vi "tdo -- V3.vi"() -> ()   [LabVIEW 2021]
uses:
  fft -- data win.ctl
  tdo -- new/Data window.ctl
  agregator -- action.ctl
  interpolation state - real.ctl
  filename-action.ctl
  <vilib>/Analysis/4window.llb/Hanning Window (DBL).vi
  <vilib>/Analysis/4window.llb/Blackman Window (DBL).vi
  linear interpolation - real -- V2.vi
  <vilib>/Analysis/4window.llb/AllCosWindow (DBL).vi
  <vilib>/Analysis/baseanly.llb/A x B.vi
  <vilib>/Analysis/baseanly.llb/Real A x B.vi
  Q -- check range -- i -- real.vi
  line -- complex.vi
  Q -- check range -- i -- integer.vi
  Q - not nan -- real.vi
  Q - not nan -- integer.vi
  <vilib>/Utility/file.llb/Write Delimited Spreadsheet (string).vi
  <vilib>/measure/matone.llb/Extract Single Tone Information 1 Chan.vi
  <vilib>/Waveform/WDTOps.llb/WDT Number of Waveform Samples DBL.vi
  <vilib>/Analysis/Matrix/Numeric/Conversions/Array To Matrix.vi
  <vilib>/Analysis/Matrix/Numeric/Conversions/Array To Matrix - RA2.vi
  <vilib>/Analysis/baseanly.llb/Inverse Matrix.vi
  <vilib>/Analysis/baseanly.llb/Real Inverse Matrix.vi
  <vilib>/Utility/file.llb/Write Delimited Spreadsheet (DBL).vi
  <vilib>/Analysis/NI_AALPro.lvlib
  <vilib>/measure/NI_MAPro.lvlib
  <vilib>/Analysis/NI_AAL_SigProc.lvlib
panel:
  in  "ccc":enum32{"Page 1", "Page 2", "Page 3"}(tab)
  in  "gamma window (sec)":dbl=0.0005 format="%#_6p"
  out "Gamma vs. Field":cluster{dbl[], dbl[]}(graph)
  out "Apmlitude or Pwr. vs. Field":cluster{dbl[], dbl[]}(graph)
  out "Frequency vs. Field":cluster{dbl[], dbl[]}(graph)
  out "Frequency vs. time":waveform(dbl)(graph)={"t0"=timestamp(-0.009969989999999984 s since 1904-01-01), "dt"=0.0001, "Y"=array[1099 elements]}
  out "Progress":dbl(slide)=0.5977589977589978 scale=0.0..1.0
  in  "aaa":enum32{"TDO settings", "file settings"}(tab)
  in  "Power spctr. threshold":dbl=0.0001 format="%.4f"
  in  "Freq. threshold":dbl=30000.0
  in  "window width (s)":dbl=0.0004 format="%#_6p"
  in  "window step (s)":dbl=0.0001 format="%#_6p"
  in  "detection method":T1(ring)
  in  "fit width":i32=9 min=3
  in  "ovewrite file?":bool
  in  "add file suffix":string="_tdo_"
  in  "remove file prefix":string="p_c4_"
  out "first line":string[](array[string])=["012_082225_time 012_082225_field 012_082225_freq 012_082225_amp 012_082225_gamma "]
  in  "Input File":path=path "/Users/arkadyshekhter/Desktop/gdrive/data/Vikram&Shiva&Zoltan--Aug2025/August_2025/082225/p_c4_012_082225.tdms"
  out "Ampl vs. time":waveform(dbl)(graph)={"t0"=timestamp(-0.009969989999999984 s since 1904-01-01), "dt"=0.0001, "Y"=array[1099 elements]}
  in  "bbb":enum32{"data settings", "Field  Settings"}(tab)
  in  "Data window":T2={"Start"=0, "Length"=1000, "Channel numbers"=[0], "Channel names"=["freq", "Field"], "Group name"="p"}
  out "dt 1":dbl=3.3e-07 format="%#_6p"
  out "dt 2":dbl=3.3e-07 format="%#_6p"
  out "Amplitude vs. Field (PWR peak)":cluster{dbl[], "Filtered X":dbl[]}(graph)
  in  "# of threads":i32=4
  out "Field profile":waveform(dbl)(graph)={"t0"=timestamp(-0.009969989999999984 s since 1904-01-01), "dt"=0.0001, "Y"=array[1099 elements]}
  # "Basic NHMFL TDO routine\nv. 0.5       F. F. Balakirev\n\nmessed with by Arkady!"
  # "Background file is either an ASCII *.dat file produced by TDO earlier\nor *.fit file containing single column of polynomial fit coeficients.\n1st row in fit file is a text header, which is ingnored. Result is saved in a \n\"*diff.dat\" file in the output folder\nExample \"PDO1.fit\": \n\nFit y=A_i*x^i, starting with A_0\n3.25637E7\n2132.56863\n-12.60591\n-2.01013\n-0.04452\n-3.23119E-4"
  # "OR"
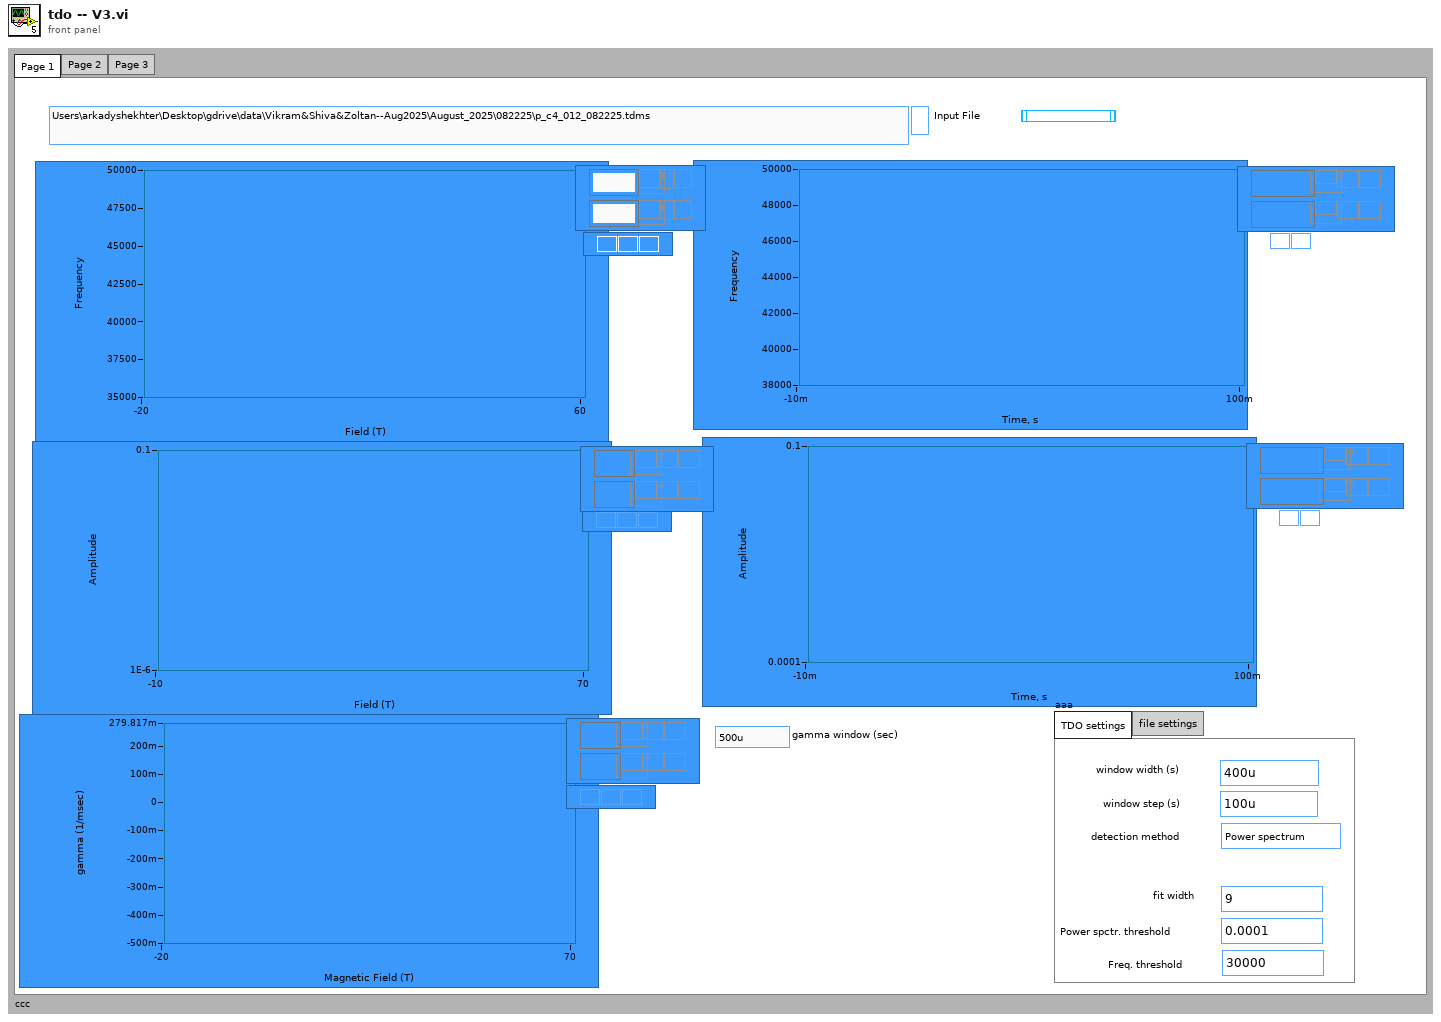
[diagram p1: front panel]
types:
  T1 = enum16{"Power spectrum", "Tone detection", "Peak-to-peak fit"}
  T2 = typedef "fft -- data win.ctl" = cluster{"Start":i64, "Length":i32, "Channel numbers":i64[], "Channel names":string[], "Group name":string}
  T3 = typedef "filename-action.ctl" = enum16{"rewrite", "parse", "force pattern", "uniquenum", "get T", "get B", "get ind", "get deg", "get name", "get folder", "get extension", "get basename", "get side", "get setof", "getID", "getIDStock", "remove prefix", "get36thing", "getplain", "getvproj", "getIDStanf"}
  T4 = typedef "interpolation state - real.ctl" = cluster{"Array ":dbl[], "actual size":i32, "requested size":i32}
  T5 = typedef "agregator -- action.ctl" = enum16{"append", "interpolate", "empty!", "force", "init", "scale", "read last"}
  T6 = typedef "Data window.ctl" = cluster{"Start":i64, "Length":i64, "Channel numbers":i64[], "Channel name":string, "Group name":string}
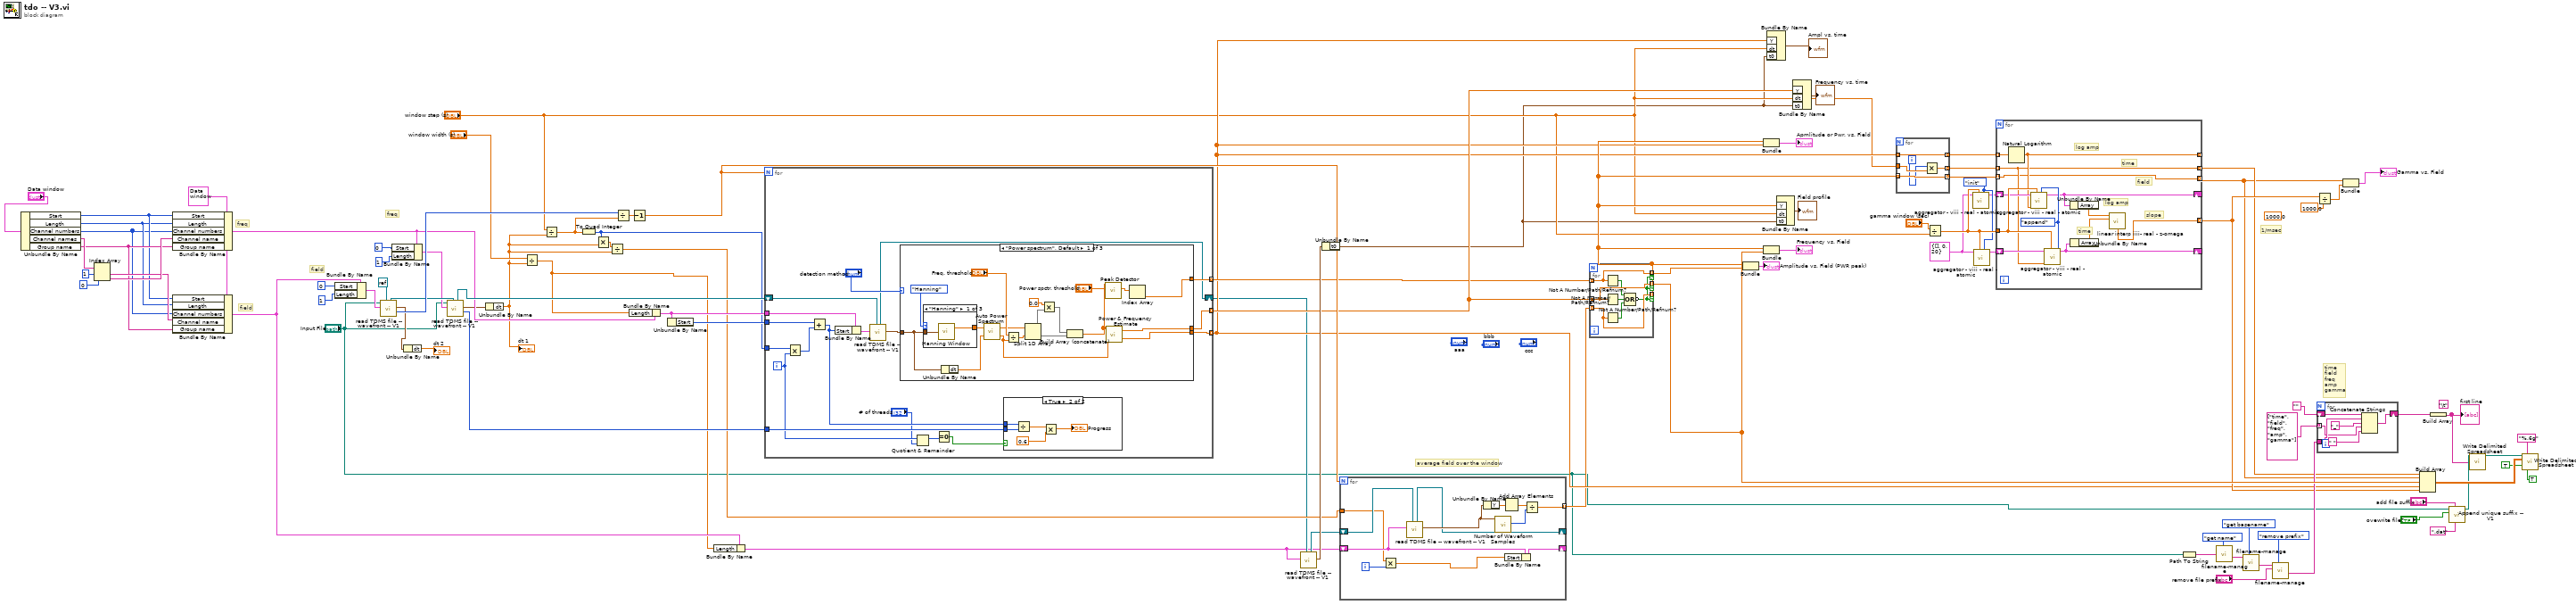
[diagram p0: block diagram]
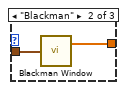
[diagram p3: hidden frame]
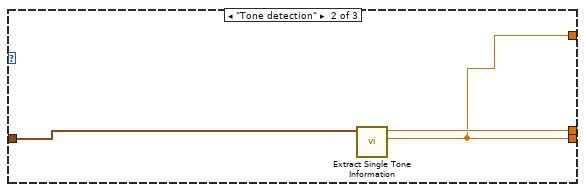
[diagram p5: hidden frame]
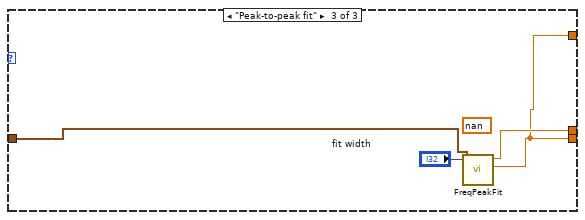
[diagram p6: hidden frame]
diagram:
  (unwired) 1000.0
  (unwired) "\t"
  w47 = T4 {"Array "=[], "actual size"=0, "requested size"=20} ("state IN")
  w51 = agregator_--_action."init" ("aggregator action")
  w14 = T6 {"Start"=0, "Length"=500000, "Channel numbers"=[0], "Channel name"="", "Group name"="Untitled"} ("Data window")
  # "average field over the window"
  # "freq"
  # "field"
  # "freq"
  # "field"
  # "1/msec"
  # "time \nfield\nfreq\namp\ngamma"
  n1 = Unbundle By Name("Data window") -> ("Start"=w11:i64, "Length"=w10:i32, "Channel numbers"=w9:i64[], "Channel names"=w81:string[], "Group name"=w12:string)
  n2 = Index Array(array=w81, index #1=1 ("index"), index #2=0 ("index")) -> (element #1=w13:string, element #2=w84:string)
  n3 = Bundle By Name(cluster=w14, "Start"=w11, "Length"=w10, "Channel numbers"=w9, "Channel name"=w84, "Group name"=w12) -> (w82:T6)
  n4 = Bundle By Name(cluster=w14, "Start"=w11, "Length"=w10, "Channel numbers"=w9, "Channel name"=w13, "Group name"=w12) -> (w8:T6)
  n5 = Bundle By Name(cluster=w8, "Start"=i64 0, "Length"=i64 1) -> (w78:T6)
  n6 = call "read TDMS file -- wavefront -- V1.vi"("tdms file in"=refnum<k0> refnum, "Data window"=w78, "Input file path"="Input File") -> ("1st channel length"=w91:u64, "Data out"=w80:waveform(dbl), "tdms file out"=w86:refnum<k34>)  [unwired: 5 in, 1 out]
  n7 = Bundle By Name(cluster=w82, "Start"=i64 0, "Length"=i64 1) -> (w77:T6)
  n8 = Unbundle By Name(w80) -> ("dt"=→"dt 2":dbl)
  n9 = call "read TDMS file -- wavefront -- V1.vi"("tdms file in"=w86, "Data window"=w77, "Input file path"="Input File") -> ("1st channel length"=w90:u64, "Data out"=w79:waveform(dbl), "tdms file out"=w87:refnum<k34>)  [unwired: 5 in, 1 out]
  n10 = Unbundle By Name(w79) -> ("dt"=w6:dbl)
  "dt 1" <- w6
  n11 = Divide(x="window width (s)", y=w6) -> (x/y=w5:dbl)
  n12 = Divide(x="window step (s)", y=w6) -> (x/y=w4:dbl)
  n13 = To Quad Integer(1:w4) -> (0:w63:i64)
  n14 = Multiply(x=w63, y=w6) -> (x*y=w62:dbl)
  n15 = Divide(x=w62, y=w6) -> (x/y=w61:dbl)
  n16 = Divide(x=w91, y=w4) -> (x/y=w76:dbl)
  n17 = Bundle By Name(cluster=w82, "Length"=w5) -> (w65:T6)
  n18 = Decrement(x=w76) -> (x-1=w68:dbl)
  n19 = Unbundle By Name(w65) -> ("Start"=w64:i64)
  n20 = Bundle By Name(cluster=w8, "Length"=w5) -> (w2:T6)
  n21 = for {
    N: w68 -> [_]
    tunnel: [w110] -> w60 mode=indexing
    tunnel: [w112] -> w25 mode=indexing
    tunnel: [w111] -> w59 mode=indexing
    tunnel: w63 -> [w107]
    tunnel: w90 -> [w109]
    tunnel: w65 -> [w106]
    tunnel: w64 -> [w105]
    shift-right: [w96] -> w17
    shift-left: w87 -> [w98]
    i -> [w101]
    n22 = Multiply(x=w107, y=w101) -> (x*y=w102:i64)
    n23 = Add(x=w105, y=w102) -> (x+y=w103:i64)
    n24 = Bundle By Name(cluster=w106, "Start"=w103) -> (w104:T6)
    n25 = call "read TDMS file -- wavefront -- V1.vi"("tdms file in"=w98, "Data window"=w104) -> ("Data out"=w108:waveform(dbl), "tdms file out"=w96:refnum<k34>)  [unwired: 6 in, 2 out]
    n26 = case shown="\"Power spectrum\", Default" "detection method" {
      tunnel: [w134 w141 w144] -> w112
      tunnel: [w122 w141 w144] -> w111
      tunnel: w108 -> [w133 w142 w147]
      tunnel: [w124 w143 w146] -> w110
      frame "Power spectrum", Default {
        n27 = case shown="\"Hanning\"" enum16{"Hanning", "Box", "Blackman"}."Hanning" ("window type") {
          tunnel: [w137 w139 w140] -> w135
          tunnel: w133 -> [w136 w138 w140]
          frame "Hanning" {
            n28 = call-poly <vilib>:"Hanning Window.vi"("X"=w136) -> ("Windowed X"=w137:dbl[])  [unwired: 1 out]
          }
          frame "Blackman" {
            n29 = call-poly <vilib>:"Blackman Window.vi"("X"=w138) -> ("Windowed X"=w139:dbl[])  [unwired: 1 out]
          }
          frame "Box" {
          }
        }
        n30 = Unbundle By Name(w133) -> ("dt"=w132:dbl)
        n31 = call <vilib>:"Auto Power Spectrum.vi"("dt"=w132, "Signal (V)"=w135) -> ("df"=w123:dbl, "Power Spectrum (V^2 rms)"=w130:dbl[])
        n32 = Divide(x="Freq. threshold", y=w123) -> (x/y=w129:dbl)
        n33 = Split 1D Array(array=w130, index=w129) -> (first subarray=w126:dbl[], second subarray=w128:dbl[])
        n34 = Multiply(x=0.0 ("element"), y=w126) -> (x*y=w125:dbl[])
        n35 = Build Array (concatenate)(w125, w128) -> (w121:dbl[])
        n36 = call <vilib>:"Peak Detector.vi"("threshold"="Power spctr. threshold", "X"=w121) -> ("Amplitudes"=w119:dbl[])  [unwired: 5 in, 4 out]
        n37 = call <vilib>:"Power & Frequency Estimate.vi"("df"=w123, "Power Spectrum (V^2 rms)"=w121) -> ("est power peak"=w134:dbl, "est frequency peak"=w124:dbl)  [unwired: 3 in, 1 out]
        n38 = Index Array(array=w119) -> (element=w122:dbl)  [unwired: 1 in]
      }
      frame "Tone detection" {
        n39 = call-poly <vilib>:"Extract Single Tone Information.vi"("time signal in"=w142) -> ("detected amplitude"=w141:dbl, "detected frequency"=w143:dbl)  [unwired: 3 in, 6 out]
      }
      frame "Peak-to-peak fit" {
        (unwired) nan
        n40 = call "FreqPeakFit.vi"("Peak fit width"="fit width", "Waveform"=w147) -> ("Amplitude"=w144:dbl, "PeakFreqOut"=w146:dbl)  [unwired: 1 in, 5 out]
      }
    }
    n41 = Quotient & Remainder(x=w101, y="# of threads") -> (x-y*floor(x/y)=w100:i32)  [unwired: 1 out]
    n42 = Equal To 0?(x=w100) -> (x = 0?=w99:bool)
    n43 = case shown="True" w99 {
      tunnel: w109 -> [_ w117]
      tunnel: w103 -> [_ w114]
      frame False {
      }
      frame True {
        n44 = Divide(x=w114, y=w117) -> (x/y=w116:dbl)
        n45 = Multiply(x=w116, y=0.6) -> (x*y=→"Progress":dbl)
      }
    }
  }
  n46 = call "read TDMS file -- wavefront -- V1.vi"("tdms file in"=w17, "Data window"=w2) -> ("Data out"=w67:waveform(dbl), "tdms file out"=w66:refnum<k34>)  [unwired: 6 in, 2 out]
  n47 = Unbundle By Name(w67) -> ("t0"=w23:timestamp)
  n48 = for {
    N: w68 -> [_]
    shift-right: [w159] -> _
    shift-left: w2 -> [w158]
    tunnel: w61 -> [w152]
    tunnel: [w157] -> w3 mode=indexing
    shift-right: [w154] -> _
    shift-left: w66 -> [w155]
    i -> [w153]
    n49 = Multiply(x=w152, y=w153) -> (x*y=w151:dbl)
    n50 = call "read TDMS file -- wavefront -- V1.vi"("tdms file in"=w155, "Data window"=w158) -> ("Data out"=w156:waveform(dbl), "tdms file out"=w154:refnum<k34>)  [unwired: 6 in, 2 out]
    n51 = Unbundle By Name(w156) -> ("Y"=w150:dbl[])
    n52 = call-poly <vilib>:"Number of Waveform Samples.vi"("waveform in"=w156) -> ("number of samples"=w149:i32)  [unwired: 1 in, 9 out]
    n53 = Add Array Elements(numeric array=w150) -> (sum=w148:dbl)
    n54 = Bundle By Name(cluster=w158, "Start"=w151) -> (w159:T6)
    n55 = Divide(x=w148, y=w149) -> (x/y=w157:dbl)
  }
  n56 = for {
    tunnel: w60 -> [w165] mode=indexing
    tunnel: w3 -> [w164] mode=indexing
    tunnel: w59 -> [w166] mode=indexing
    tunnel: [w166] -> w57 mode=indexing if=w160
    tunnel: [w165] -> w58 mode=indexing if=w160
    tunnel: [w164] -> w55 mode=indexing if=w160
    n57 = Not A Number/Path/Refnum?(number/path/refnum=w166) -> (NaN/Path/Refnum?=w163:bool)
    n58 = Not A Number/Path/Refnum?(number/path/refnum=w165) -> (NaN/Path/Refnum?=w162:bool)
    n59 = Not A Number/Path/Refnum?(number/path/refnum=w164) -> (NaN/Path/Refnum?=w161:bool)
    n60 = Compound Arithmetic op=OR(w163, w162, w161) -> (invert w160:bool)
  }
  n61 = Bundle(w55, w57) -> (→"Amplitude vs. Field (PWR peak)":cluster{dbl[], dbl[]})  [unwired: 1 out]
  n62 = Bundle(w55, w25) -> (→"Apmlitude or Pwr. vs. Field":cluster{dbl[], dbl[]})  [unwired: 1 out]
  n63 = Bundle(w55, w58) -> (→"Frequency vs. Field":cluster{dbl[], dbl[]})  [unwired: 1 out]
  n64 = Bundle By Name("Y"=w25, "dt"="window step (s)", "t0"=w23) -> (→"Ampl vs. time":waveform(dbl))  [unwired: 1 out]
  n65 = Bundle By Name("Y"=w55, "dt"="window step (s)", "t0"=w23) -> (→"Field profile":waveform(dbl))  [unwired: 1 out]
  n66 = Bundle By Name("Y"=w60, "dt"="window step (s)", "t0"=w23) -> (→"Frequency vs. time":waveform(dbl))  [unwired: 1 out]
  n67 = for {
    tunnel: w25 -> [w169] mode=indexing
    tunnel: "window step (s)" -> [w171]
    tunnel: [w170] -> w46 mode=indexing
    tunnel: [w169] -> w53 mode=indexing
    tunnel: [w168] -> w49 mode=indexing
    tunnel: w55 -> [w168] mode=indexing
    i -> [w167]
    n68 = Multiply(x=w167, y=w171) -> (x*y=w170:dbl)
  }
  n69 = Divide(x="gamma window (sec)", y="window step (s)") -> (x/y=w52:dbl)
  n70 = call "aggregator - viii - real - atomic.vi"("aggregator action"=w51, "requested size"=w52, "state IN"=w47) -> ("state OUT"=w50:T4)  [unwired: 5 in, 3 out]
  n71 = call "aggregator - viii - real - atomic.vi"("aggregator action"=w51, "requested size"=w52, "state IN"=w47) -> ("state OUT"=w54:T4)  [unwired: 5 in, 3 out]
  n72 = for {
    shift-right: [w178] -> _
    shift-left: w54 -> [w184]
    tunnel: w52 -> [w181]
    tunnel: w53 -> [w183] mode=indexing
    tunnel: w46 -> [w173] mode=indexing
    shift-right: [w179] -> _
    shift-left: w50 -> [w180]
    tunnel: [w175] -> w27 mode=indexing
    tunnel: [w174] -> _ mode=indexing
    tunnel: [w173] -> w19 mode=indexing
    tunnel: w49 -> [w172] mode=indexing
    tunnel: [w172] -> w18 mode=indexing
    w182 = agregator_--_action."append" ("aggregator action")
    # "field"
    # "slope"
    # "time"
    # "log amp"
    # "log amp"
    # "time"
    n73 = Natural Logarithm(1:w183) -> (0:w174:dbl)
    n74 = call "aggregator - viii - real - atomic.vi"("aggregator action"=w182, "requested size"=w181, "number"=w174, "state IN"=w180) -> ("state OUT"=w179:T4)  [unwired: 4 in, 3 out]
    n75 = call "aggregator - viii - real - atomic.vi"("aggregator action"=w182, "requested size"=w181, "number"=w173, "state IN"=w184) -> ("state OUT"=w178:T4)  [unwired: 4 in, 3 out]
    n76 = Unbundle By Name(w179) -> ("Array"=w176:dbl[])
    n77 = Unbundle By Name(w178) -> ("Array"=w177:dbl[])
    n78 = call "linear interp iiii- real - z-omega.vi"("z"=w176, "omega"=w177) -> ("slope"=w175:dbl)  [unwired: 4 in, 9 out]
  }
  n79 = Path To String(path="Input File") -> (string=w36:string)
  n80 = call "filename-manage.vi"("filename-action"=filename-action."get name", "file name IN"=w36) -> ("string OUT"=w35:string)  [unwired: 7 in, 2 out]
  n81 = call "filename-manage.vi"("filename-action"=filename-action."get basename", "file name IN"=w35) -> ("string OUT"=w33:string)  [unwired: 7 in, 2 out]
  n82 = call "filename-manage.vi"("filename-action"=filename-action."remove prefix", "string IN"="remove file prefix", "file name IN"=w33) -> ("string OUT"=w30:string)  [unwired: 6 in, 2 out]
  n83 = Divide(x=w27, y=1000.0) -> (x/y=w26:dbl[])
  n84 = for {
    tunnel: string[] ["time", "field", "freq", "amp", "gamma"] -> [w186] mode=indexing
    shift-right: [w189] -> w28
    shift-left: "" ("format (%.3f)") -> [w190]
    tunnel: w30 -> [w188]
    n85 = Concatenate Strings(w190, w188, "_", w186, " ") -> (w189:string)
  }
  n86 = Bundle(w18, w26) -> (→"Gamma vs. Field":cluster{dbl[], dbl[]})  [unwired: 1 out]
  n87 = Build Array(w19, w18, w58, w25, w27) -> (w74:dbl[][])
  n88 = Build Array(w28) -> (w39:string[])
  "first line" <- w39
  n89 = call "Append unique suffix -- V1.vi"("Extention"=".dat", "Suffix"="add file suffix", "ovewrite ?"="ovewrite file?", "Path"="Input File") -> ("Path out"=w40:path)  [unwired: 6 in, 1 out]
  n90 = call-poly <vilib>:"Write Delimited Spreadsheet.vi"("file path (dialog if empty)"=w40, "1D data"=w39) -> ("new file path (Not A Path if cancelled)"=w38:path)  [unwired: 12 in, 1 out]
  n91 = call-poly <vilib>:"Write Delimited Spreadsheet.vi"("file path (dialog if empty)"=w38, "format (%.3f)"="%.6g", "2D data"=w74, "append to file? (new file:F)"=TRUE, "transpose? (no:F)"=TRUE) -> ()  [unwired: 9 in, 2 out]
